vi "Read Configuration Parameters.vi"(8 "error in (no error)":errorcluster, 10 "refnum":T1, 11 "Step Configuration in":refnum<class "Step Configuration.lvclass">) -> (0 "error out":errorcluster, 2 "refnum out":T1, 3 "Step Configuration out":refnum<class "Step Configuration.lvclass">)   [LabVIEW 2026, in "Measurement Actor.lvlib" / "Step Configuration.lvclass"]
uses:
  Step Configuration.lvclass
  C:/Users/E2013170/Documents/GitHub/Measurement-Utility-Reference/components/Extensible-Config-Dialog/Configuration.lvclass
  <vilib>/Utility/config.llb/Config Data RefNum.ctl
  Extensible-Config-Dialog/Configuration.lvclass/Configuration.ctl
  Step Configuration.lvclass/Step Configuration.ctl
  Extensible-Config-Dialog/Configuration.lvclass
  Logger/config/Logger Configuration.lvclass
  <vilib>/Utility/config.llb/NI_LVConfig.lvlib
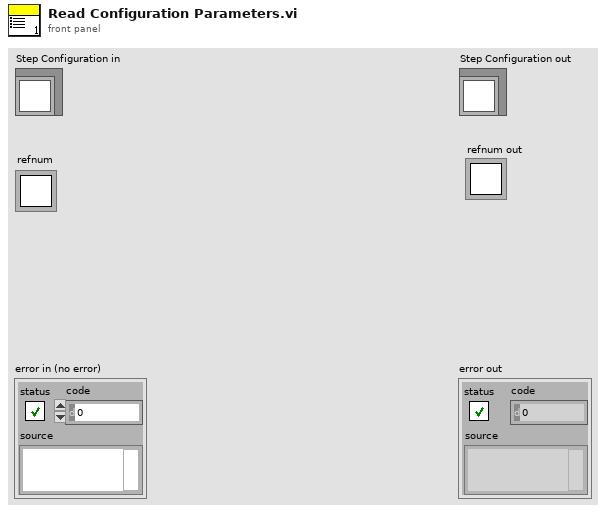
[diagram p1: front panel]
types:
  T1 = typedef "NI_LVConfig.lvlib/Config Data RefNum.ctl" = refnum<k1>
  T2 = cluster{"Run indefinitely":bool, "Iterations":i32}
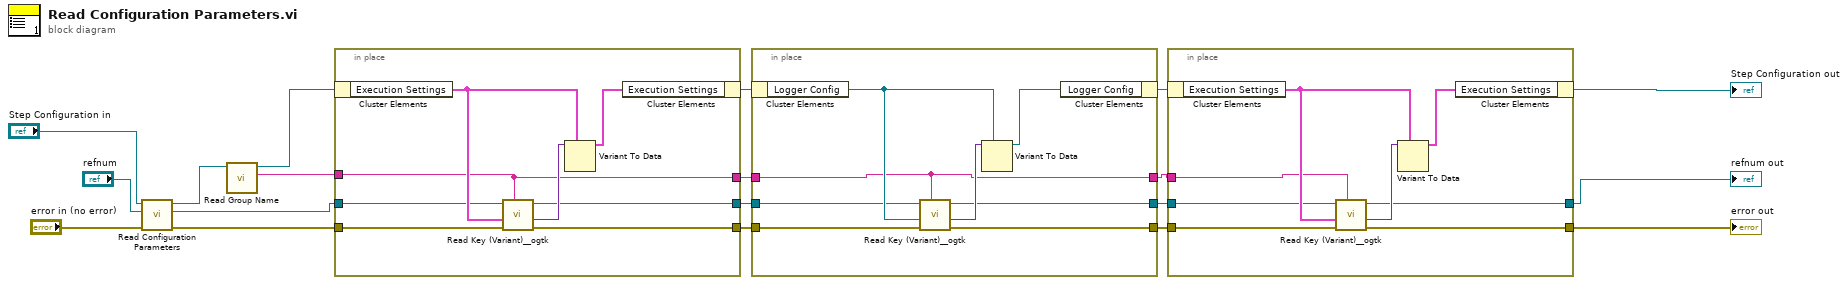
[diagram p0: block diagram]
diagram:
  n1 = call-parent "Read Configuration Parameters.vi"("error in (no error)"="error in (no error)", "refnum"="refnum", "Configuration in"="Step Configuration in") -> ("error out"=w15:errorcluster, "refnum out"=w16:T1, "Configuration out"=w14:refnum<class "Step Configuration.lvclass">)  [unwired: 6 in]
  n2 = call "Read Group Name.vi"("Configuration in"=w14) -> ("Group Name"=w9:string, "Configuration out"=w10:refnum<class "Step Configuration.lvclass">)  [unwired: 8 in, 1 out]
  n3 = in-place {
    in-place-border: w16 -> [w24]
    in-place-border: [w23] -> w13
    in-place-border: w15 -> [w22]
    in-place-border: [w21] -> w12
    in-place-border: w9 -> [w20]
    in-place-border: [w20] -> w8
    n4 = in-place-cluster #1(w10) -> ("Execution Settings"=w27:T2)
    n5 = call "Read Key (Variant)__ogtk.vi"("section"=w20, "error in (no error)"=w22, "type"=w27, "refnum"=w24) -> ("error out"=w21:errorcluster, "key-value"=w26:variant, "refnum out"=w23:T1)  [unwired: 4 in, 1 out]
    n6 = Variant To Data(type=w27, Variant=w26) -> (data=w25:T2)  [unwired: 1 in, 1 out]
    n7 = in-place-cluster #1("Execution Settings"=w25) -> (w11:refnum<class "Step Configuration.lvclass">)
  }
  n8 = in-place {
    in-place-border: w13 -> [w32]
    in-place-border: [w31] -> w5
    in-place-border: w12 -> [w30]
    in-place-border: [w29] -> w4
    in-place-border: w8 -> [w28]
    in-place-border: [w28] -> w6
    n9 = in-place-cluster #2(w11) -> ("Logger Config"=w35:refnum<class "Logger Configuration.lvclass">)
    n10 = call "Read Key (Variant)__ogtk.vi"("section"=w28, "error in (no error)"=w30, "type"=w35, "refnum"=w32) -> ("error out"=w29:errorcluster, "key-value"=w34:variant, "refnum out"=w31:T1)  [unwired: 4 in, 1 out]
    n11 = Variant To Data(type=w35, Variant=w34) -> (data=w33:refnum<class "Logger Configuration.lvclass">)  [unwired: 1 in, 1 out]
    n12 = in-place-cluster #2("Logger Config"=w33) -> (w7:refnum<class "Step Configuration.lvclass">)
  }
  n13 = in-place {
    in-place-border: w5 -> [w40]
    in-place-border: [w39] -> w2
    in-place-border: w4 -> [w38]
    in-place-border: [w37] -> w3
    in-place-border: w6 -> [w36]
    n14 = in-place-cluster #3(w7) -> ("Execution Settings"=w43:T2)
    n15 = call "Read Key (Variant)__ogtk.vi"("section"=w36, "error in (no error)"=w38, "type"=w43, "refnum"=w40) -> ("error out"=w37:errorcluster, "key-value"=w42:variant, "refnum out"=w39:T1)  [unwired: 4 in, 1 out]
    n16 = Variant To Data(type=w43, Variant=w42) -> (data=w41:T2)  [unwired: 1 in, 1 out]
    n17 = in-place-cluster #3("Execution Settings"=w41) -> (→"Step Configuration out":refnum<class "Step Configuration.lvclass">)
  }
  "error out" <- w3
  "refnum out" <- w2
